vi "Desktop Execution - Generate Trace Events.vi"() -> ()   [LabVIEW 2023]
doc: "This example shows how to generate events that can be traced using the <B>Desktop Execution Trace Toolkit</B>."
panel:
  out "Initialized array":u32[](array[numeric])
  in  "Trace Event Structure Cases":bool
  in  "Queues (Blocked)":bool
  in  "Notifiers":bool
  in  "Select, drag, and drop me":string="Select, drag, and drop me"
  in  "Memory Allocations":bool
  in  "Timeout (ms)":i32=-1
  in  "User Events":u16(ring) items=["generate"]
  in  "Test User String":string="Test User String"
  in  "Errors":bool
  in  "User-Defined Trace Events":bool
  in  "Close the reference after loading a dynamic VI":bool
  in  "Stop":bool
  in  "Load Dynamic VI":bool
  in  "Queues":bool
  in  "OK":bool
  # "Overview: Demonstrates the types of events that the Desktop Execution Trace Toolkit can trace.\nRequirements: Desktop Execution Trace Toolkit\nInstructions:\nNote: If you open this example by following the Getting Started section in the LabVIEW Desktop Execution Trace Toolkit for Windows Help, skip the following steps.\n1.\tLaunch the Desktop Execution Trace Toolkit by selecting Tools>>Profile>>Trace Execution from the LabVIEW menu bar.\n2.\tSelect Tools>>Options from the LabVIEW menu bar and select VI Server from the Category list to enable VI Server support and machine access.\n3.\tIn the Desktop Execution Trace Toolkit, click the lower part of the Capture Settings button and select the Memory Allocations checkbox from the Capture Settings pull-down menu.\n4.\tClick Start on the Home tab.\n5.\tIn LabVIEW, run the VI. Click the buttons on the front panel to generate different types of events for the Desktop Execution Trace Toolkit to capture. You can review the events in the Desktop Execution Trace Toolkit."
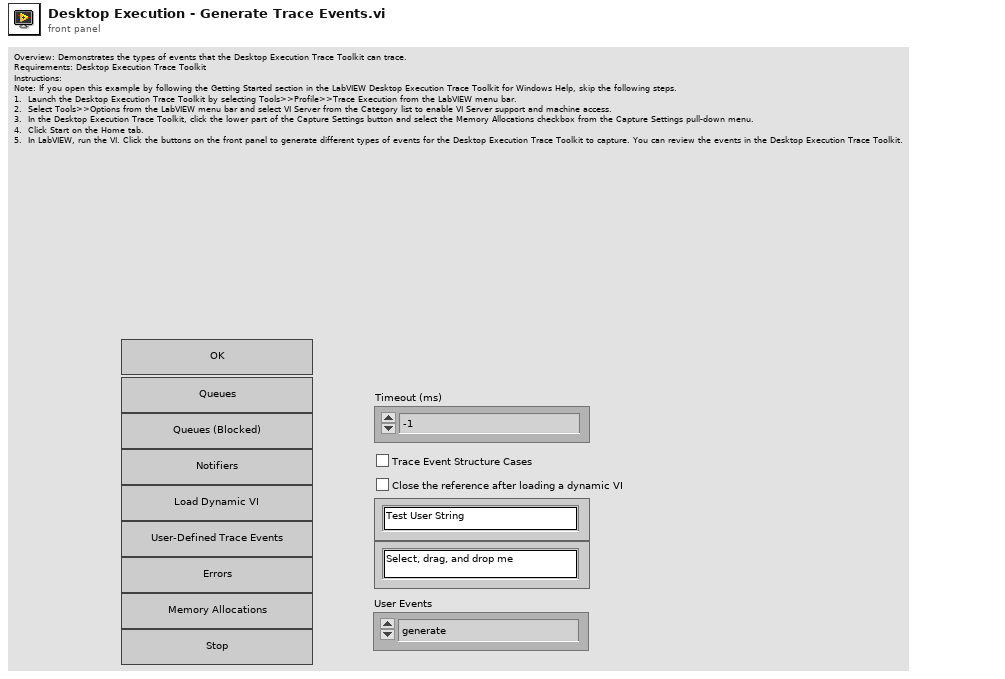
[diagram p1: front panel]
types:
  T1 = enum32{"Invalid", "Standard", "Closed", "Hidden", "Minimized", "Maximized"}
  T2 = enum16{"open", "replace", "create", "open or create", "replace or create", "replace or create with confirmation"}
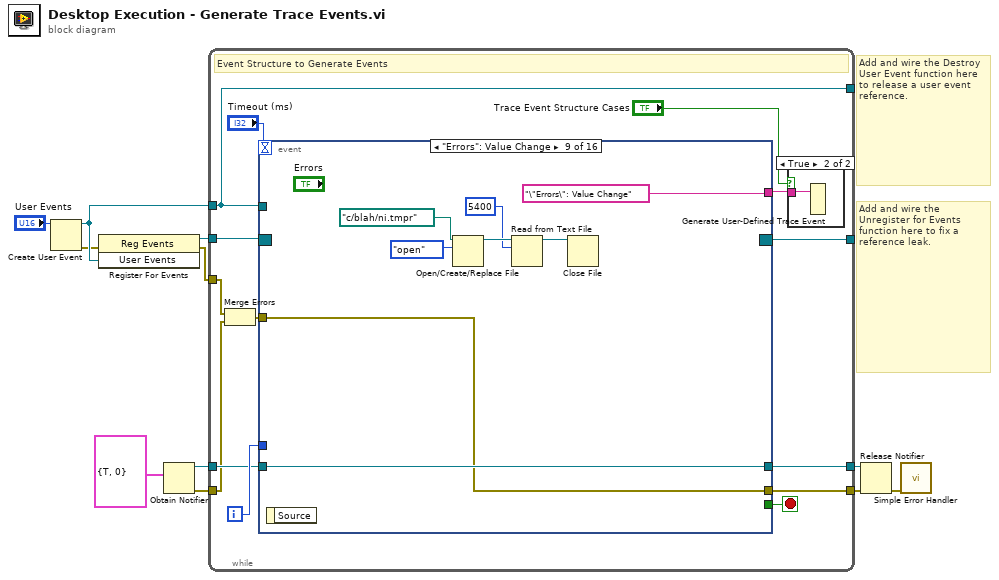
[diagram p0: block diagram]
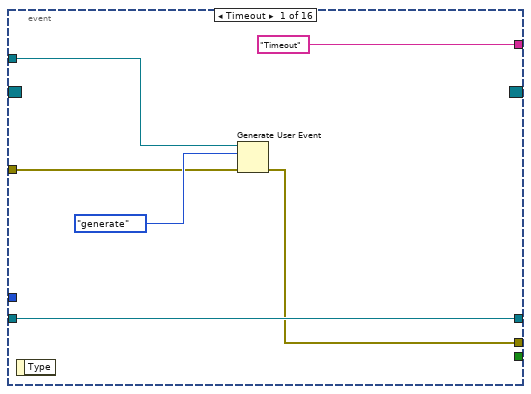
[diagram p3: hidden frame]
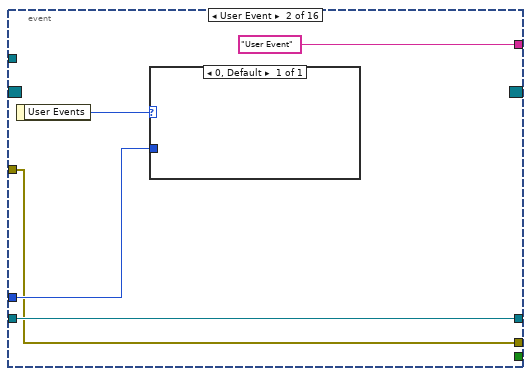
[diagram p4: hidden frame]
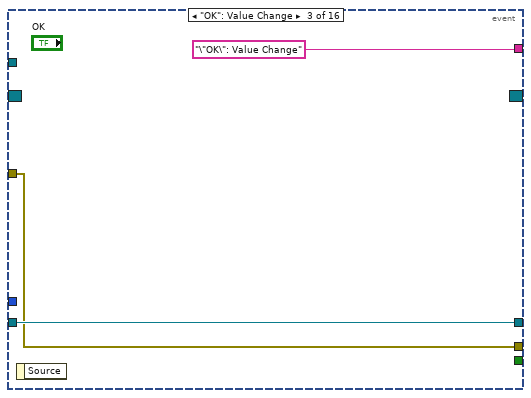
[diagram p5: hidden frame]
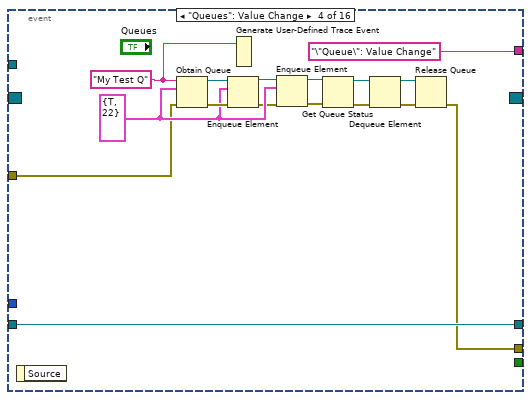
[diagram p6: hidden frame]
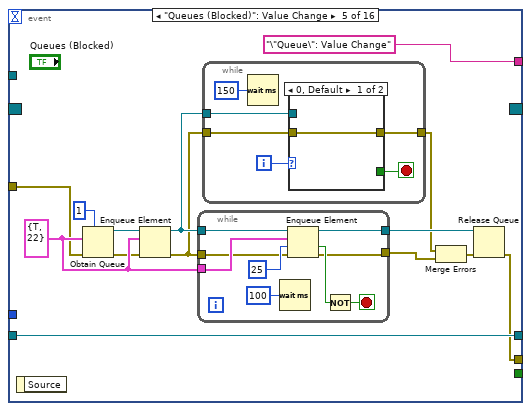
[diagram p7: hidden frame]
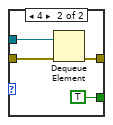
[diagram p8: hidden frame]
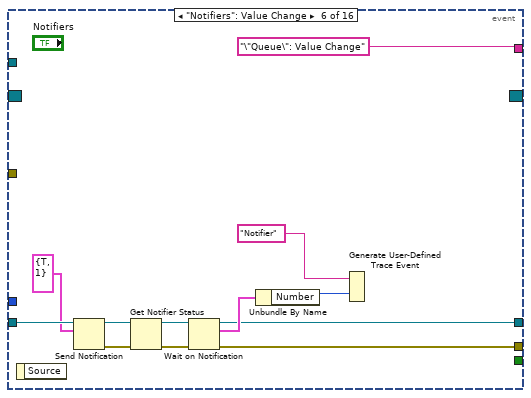
[diagram p9: hidden frame]
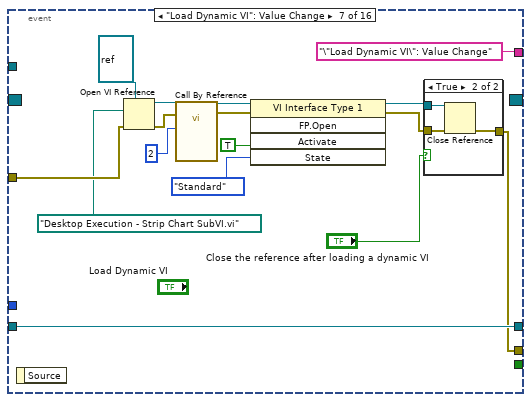
[diagram p10: hidden frame]
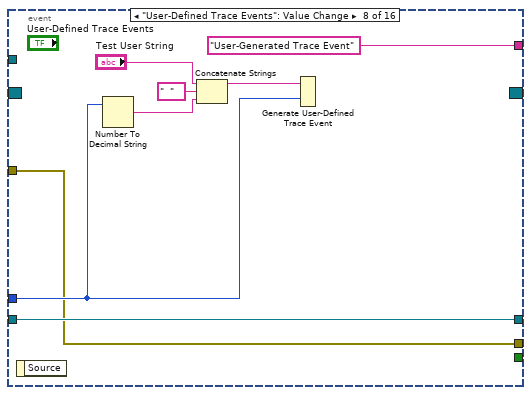
[diagram p12: hidden frame]
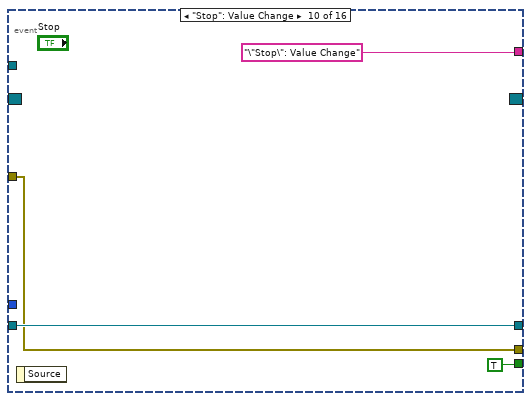
[diagram p13: hidden frame]
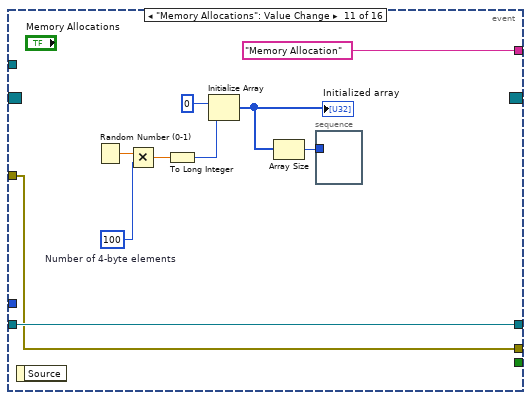
[diagram p14: hidden frame]
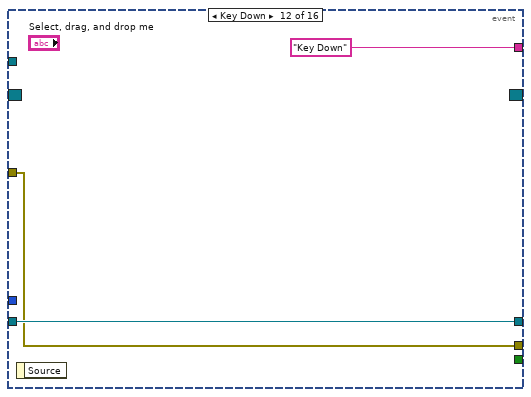
[diagram p15: hidden frame]
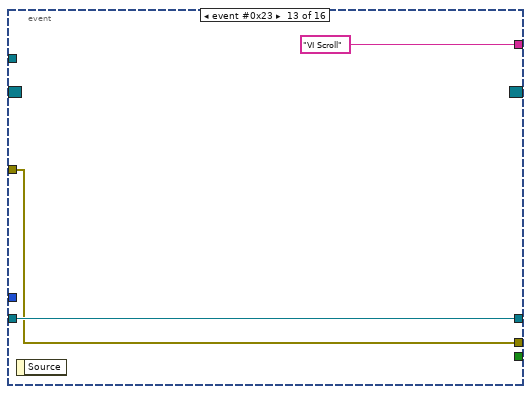
[diagram p16: hidden frame]
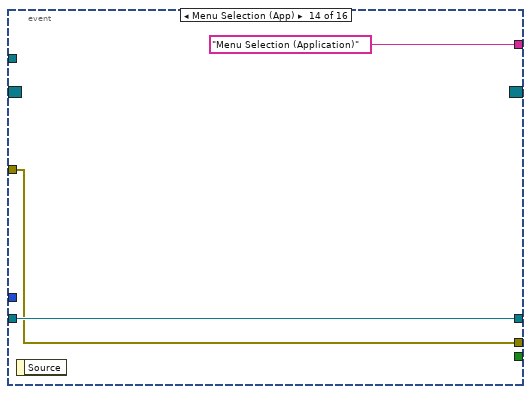
[diagram p17: hidden frame]
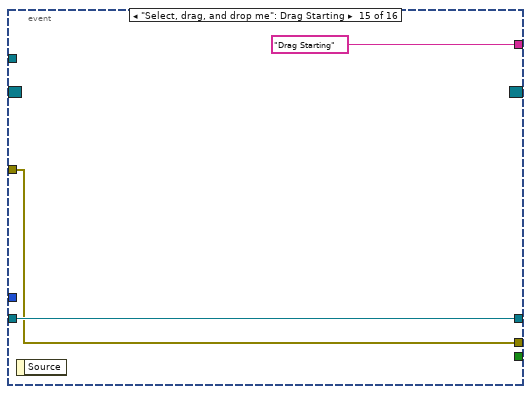
[diagram p18: hidden frame]
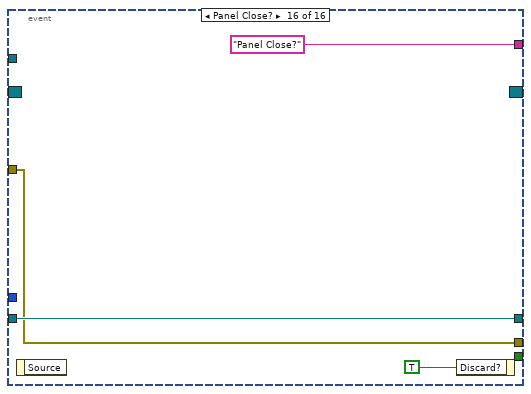
[diagram p19: hidden frame]
diagram:
  # "Add and wire the Destroy User Event function here to release a user event reference."
  # "Add and wire the Unregister for Events function here to fix a reference leak."
  n1 = Create User Event(user event datatype="User Events") -> (user event=w9:refnum<user-event>, error out=w5:errorcluster)  [unwired: 1 in]
  n2 = register-events(error in=w5, w9) -> (reference out=w10:refnum<event-registration>, error out=w4:errorcluster)  [unwired: 1 in]
  n3 = Obtain Notifier(notification data type=cluster{"Bool":bool, "Number":i32} {"Bool"=TRUE, "Number"=0}) -> (notifier out=w7:refnum<notifier>, error out=w3:errorcluster)  [unwired: 2 in, 2 out]
  n4 = while {
    tunnel: w10 -> [w24]
    tunnel: w9 -> [w23]
    tunnel: [w23] -> _
    tunnel: [w22] -> _
    tunnel: w7 -> [w20]
    tunnel: [w19] -> w6
    tunnel: w4 -> [w15]
    tunnel: w3 -> [w16]
    tunnel: [w13] -> w2
    i -> [w25]
    stop <- w12 stop-if-true
    # "Event Structure to Generate Events"
    n5 = Merge Errors(w15, w16) -> (w14:errorcluster)
    n6 = event shown="[8] \"Errors\": Value Change" {
      selector: w24 -> [_ _ _ _ _ _ _ _ _ _ _ _ _ _ _ _]
      dyn-events: [_ _ _ _ _ _ _ _ _ _ _ _ _ _ _ _] -> w22
      timeout: "Timeout (ms)" -> [_ _ _ _ _ _ _ _ _ _ _ _ _ _ _ _]
      tunnel: [_ _ _ _ _ _ _ _ _ TRUE _ _ _ _ _ _] -> w12
      tunnel: w25 -> [_ w36 _ _ _ _ _ w126 _ _ _ _ _ _ _ _]
      tunnel: w23 -> [w28 _ _ _ _ _ _ _ _ _ _ _ _ _ _ _]
      tunnel: ["Timeout" "User Event" "\"OK\": Value Change" "\"Queue\": Value Change" "\"Queue\": Value Change" "\"Queue\": Value Change" "\"Load Dynamic VI\": Value Change" "User-Generated Trace Event" "\"Errors\": Value Change" "\"Stop\": Value Change" "Memory Allocation" "Key Down" "VI Scroll" "Menu Selection (Application)" "Drag Starting" "Panel Close?"] -> w17
      tunnel: w20 -> [w31 w35 w39 w47 w70 w101 w113 w125 w132 w140 w150 w155 w158 w161 w164 w168]
      tunnel: [w31 w35 w39 w47 w70 w94 w113 w125 w132 w140 w150 w155 w158 w161 w164 w168] -> w19
      tunnel: w14 -> [w30 w34 w38 w43 w65 _ w110 w123 w131 w139 w143 w154 w157 w160 w163 w167]
      tunnel: [w29 w34 w38 w42 w57 w91 w111 w123 w131 w139 w143 w154 w157 w160 w163 w167] -> w13
      event Timeout {
        n7 = event-data() -> ()  [unwired: 2 out]
        n8 = Generate User Event(user event=w28, event data cluster=enum16{"generate"}."generate" ("event data"), error in=w30) -> (error out=w29:errorcluster)  [unwired: 1 in, 1 out]
      }
      event User Event {
        n9 = event-data() -> ("User Events"=w37:u16)  [unwired: 1 out]
        n10 = case shown="0, Default" w37 {
          tunnel: w36 -> [_]
          frame 0, Default {
          }
        }
      }
      event "OK": Value Change {
        n11 = event-data() -> ()  [unwired: 2 out]
      }
      event "Queues": Value Change {
        w48 = cluster{bool, i32} {TRUE, 22}
        w46 = "My Test Q" ("name (unnamed)")
        n12 = event-data() -> ()  [unwired: 2 out]
        n13 = Obtain Queue(name (unnamed)=w46, element data type=w48, error in (no error)=w43) -> (queue out=w56:refnum<queue>, error out=w54:errorcluster)  [unwired: 2 in, 1 out]
        n14 = Enqueue Element(queue=w56, element=w48, error in (no error)=w54) -> (queue out=w41:refnum<queue>, error out=w45:errorcluster)  [unwired: 2 out]
        n15 = Generate User-Defined Trace Event(2:w46) -> ()  [unwired: 1 out]
        n16 = Enqueue Element(queue=w41, element=w48, error in (no error)=w45) -> (queue out=w49:refnum<queue>, error out=w44:errorcluster)  [unwired: 2 out]
        n17 = Get Queue Status(queue=w49, error in (no error)=w44) -> (queue out=w50:refnum<queue>, error out=w51:errorcluster)  [unwired: 7 out]
        n18 = Dequeue Element(queue=w50, error in (no error)=w51) -> (queue out=w55:refnum<queue>, error out=w53:errorcluster)  [unwired: 3 out]
        n19 = Release Queue(queue=w55, error in (no error)=w53) -> (error out=w42:errorcluster)  [unwired: 3 out]
      }
      event "Queues (Blocked)": Value Change {
        w67 = cluster{bool, i32} {TRUE, 22}
        n20 = event-data() -> ()  [unwired: 2 out]
        n21 = Obtain Queue(max queue size (-1, unlimited)=1, element data type=w67, error in (no error)=w65) -> (queue out=w69:refnum<queue>, error out=w64:errorcluster)  [unwired: 1 in, 2 out]
        n22 = Enqueue Element(queue=w69, element=w67, error in (no error)=w64) -> (queue out=w68:refnum<queue>, error out=w61:errorcluster)  [unwired: 2 out]
        n23 = while {
          tunnel: w68 -> [w78]
          tunnel: w67 -> [w77]
          tunnel: [w73] -> w66
          tunnel: w61 -> [w72]
          tunnel: [w71] -> w60
          stop <- w74 stop-if-true
          n24 = Wait (ms)(milliseconds to wait=u32 100) -> ()  [unwired: 1 out]
          n25 = Enqueue Element(queue=w78, element=w77, timeout in ms (-1)=25, error in (no error)=w72) -> (queue out=w73:refnum<queue>, timed out?=w75:bool, error out=w71:errorcluster)
          n26 = Not(x=w75) -> (.not. x?=w74:bool)
        }
        n27 = while {
          tunnel: w68 -> [w82]
          tunnel: w61 -> [w81]
          tunnel: [w80] -> w58
          i -> [w84]
          stop <- w83 stop-if-true
          n28 = Wait (ms)(milliseconds to wait=u32 150) -> ()  [unwired: 1 out]
          n29 = case shown="0, Default" w84 {
            tunnel: [_ TRUE] -> w83
            tunnel: w82 -> [_ w89]
            tunnel: w81 -> [w86 w88]
            tunnel: [w86 w87] -> w80
            frame 0, Default {
            }
            frame 4 {
              n30 = Dequeue Element(queue=w89, error in (no error)=w88) -> (error out=w87:errorcluster)  [unwired: 4 out]
            }
          }
        }
        n31 = Merge Errors(w58, w60) -> (w59:errorcluster)
        n32 = Release Queue(queue=w66, error in (no error)=w59) -> (error out=w57:errorcluster)  [unwired: 3 out]
      }
      event "Notifiers": Value Change {
        n33 = event-data() -> ()  [unwired: 2 out]
        n34 = Send Notification(notification=cluster{"Bool":bool, "Number":i32} {"Bool"=TRUE, "Number"=1}, notifier=w101) -> (notifier out=w99:refnum<notifier>, error out=w98:errorcluster)  [unwired: 1 in]
        n35 = Get Notifier Status(notifier=w99, error in (no error)=w98) -> (notifier out=w93:refnum<notifier>, error out=w92:errorcluster)  [unwired: 3 out]
        n36 = Wait on Notification(notifier=w93, error in (no error)=w92) -> (notifier out=w94:refnum<notifier>, notification=w97:cluster{"Bool":bool, "Number":i32}, error out=w91:errorcluster)  [unwired: 3 out]
        n37 = Unbundle By Name(w97) -> ("Number"=w96:i32)
        n38 = Generate User-Defined Trace Event(1:w96, 2:"Notifier" ("trace string")) -> ()
      }
      event "Load Dynamic VI": Value Change {
        n39 = event-data() -> ()  [unwired: 2 out]
        n40 = Open VI Reference(type specifier VI Refnum (for type only)=refnum<vi> refnum, vi path=path "Desktop Execution - Strip Chart SubVI.vi", error in (no error)=w110) -> (vi reference=w117:refnum<vi>, error out=w112:errorcluster)  [unwired: 3 out]
        n41 = call-by-ref "?"(reference=w117, error in=w112, "Numeric"=2) -> (reference out=w109:refnum<vi>, error out=w108:errorcluster)  [unwired: 11 in]
        n42 = invoke class="VI Interface Type 1" method="FP.Open"(reference=w109, error in=w108, "Activate"=TRUE ("Activate?"), "State"=T1."Standard") -> (reference out=w106:refnum<vi>, error out=w107:errorcluster)  [unwired: 1 in, 3 out]
        n43 = case shown="True" "Close the reference after loading a dynamic VI" {
          tunnel: w106 -> [_ w122]
          tunnel: w107 -> [w119 w121]
          tunnel: [w119 w120] -> w111
          frame False {
          }
          frame True {
            n44 = Close Reference(reference=w122, error in (no error)=w121) -> (error out=w120:errorcluster)
          }
        }
      }
      event "User-Defined Trace Events": Value Change {
        n45 = event-data() -> ()  [unwired: 2 out]
        n46 = Number To Decimal String(number=w126) -> (decimal integer string=w128:string)  [unwired: 1 out]
        n47 = Concatenate Strings("Test User String", "  " ("string"), w128) -> (w127:string)
        n48 = Generate User-Defined Trace Event(1:w126, 2:w127) -> ()
      }
      event "Errors": Value Change {
        n49 = event-data() -> ()  [unwired: 2 out]
        n50 = Open/Create/Replace File(file path (use dialog)=path "c:/blah/ni.tmpr", operation (0:open)=T2."open") -> (refnum out=w136:refnum<file>)  [unwired: 1 in, 5 out]
        n51 = Read from Text File(file (use dialog)=w136, count=5400) -> (refnum out=w133:refnum<file>)  [unwired: 1 in, 4 out]
        n52 = Close File(refnum=w133) -> ()  [unwired: 1 in, 2 out]
      }
      event "Stop": Value Change {
        n53 = event-data() -> ()  [unwired: 2 out]
      }
      event "Memory Allocations": Value Change {
        w146 = 100  # Number of 4-byte elements
        n54 = event-data() -> ()  [unwired: 2 out]
        n55 = Random Number (0-1)() -> (number: 0 to 1=w147:dbl)
        n56 = Multiply(x=w147, y=w146) -> (x*y=w145:dbl)
        n57 = To Long Integer(number=w145) -> (32bit integer=w144:i32)
        n58 = Initialize Array(u32 0, w144) -> (w151:u32[])
        "Initialized array" <- w151
        n59 = Array Size(array=w151) -> (size(s)=w148:i32)
        n60 = stacked-sequence {
          tunnel: w148 -> [_]
          frame #0 {
          }
        }
      }
      event Key Down {
        n61 = event-data() -> ()  [unwired: 2 out]
      }
      event event #0x23 {
        n62 = event-data() -> ()  [unwired: 2 out]
      }
      event Menu Selection (App) {
        n63 = event-data() -> ()  [unwired: 2 out]
      }
      event "Select, drag, and drop me": Drag Starting {
        n64 = event-data() -> ()  [unwired: 2 out]
      }
      event Panel Close? {
        n65 = event-data() -> ()  [unwired: 2 out]
        n66 = event-data("Discard?"=TRUE) -> ()  [unwired: 1 in, 1 out]
      }
    }
    n67 = case shown="True" "Trace Event Structure Cases" {
      tunnel: w17 -> [_ w26]
      frame False {
      }
      frame True {
        n68 = Generate User-Defined Trace Event(2:w26) -> ()  [unwired: 1 out]
      }
    }
  }
  n69 = Release Notifier(notifier=w6, error in (no error)=w2) -> (error out=w1:errorcluster)  [unwired: 3 out]
  n70 = call <vilib>:"Simple Error Handler.vi"("error in (no error)"=w1) -> ()  [unwired: 4 in, 5 out]
